vi "Asynchronous - RT Command Channels - Execute.vi"(7 "Map (RT Command Channels)":T1[](array[typedef]) {"RT Command Channel Ref" format="%.0x"}, 8 "Error (in)":errorcluster, 11 "Changes?":bool[](array[boolean])) -> (0 "Error (out)":errorcluster)   [LabVIEW 2017, in "Ballard MIL-1553 Engine.lvlib"]
uses:
  Ballard MIL-1553 Engine.lvlib
  Controls/RT Async_Map RT Command Channels.ctl
  Controls/RT Async_Map_Type.ctl
  <vilib>/NI Veristand/Custom Device API/Custom Device Item Ref.ctl
  <instrlib>/BTI1553Lib/BTI1553LV.lvlib
  <vilib>/NI VeriStand/Custom Device Tools/Custom Device Utility Library/Custom Device Utility Library.lvlib
  <vilib>/NI VeriStand/Custom Device API/Custom Device API.lvlib
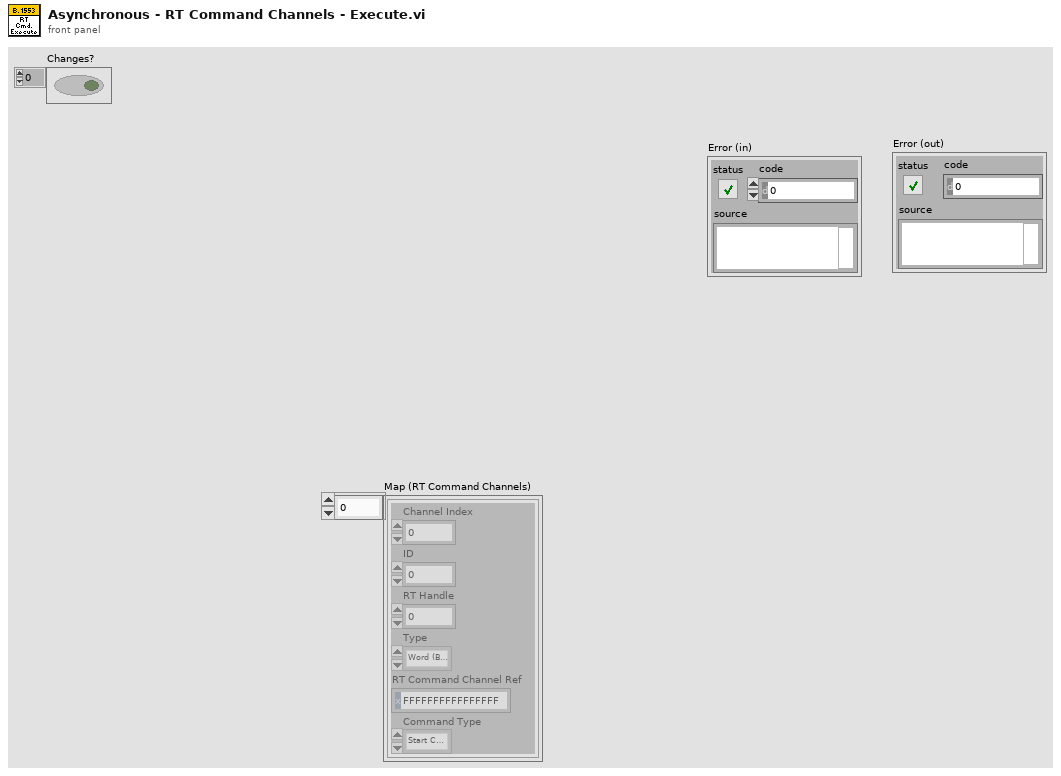
[diagram p1: front panel]
types:
  T1 = typedef "Ballard MIL-1553 Engine.lvlib/RT Async_Map RT Command Channels.ctl" = cluster{"Channel Index":i32, "ID":i32, "RT Handle":u64, "Type":T2, "RT Command Channel Ref":T3, "Command Type":enum16{"Start Command", "Stop Command"}}
  T2 = typedef "Ballard MIL-1553 Engine.lvlib/RT Async_Map_Type.ctl" = enum16{"Word (BC to RT)", "Word (MC (Rx))", "Acyclic Message Trigger", "Word (RT to ..)", "Word (RT to RT)", "Word (MC (Tx))", "RT Status", "BC Commands", "RT Commands"}
  T3 = typedef "Custom Device API.lvlib/Custom Device Item Ref.ctl" = u64
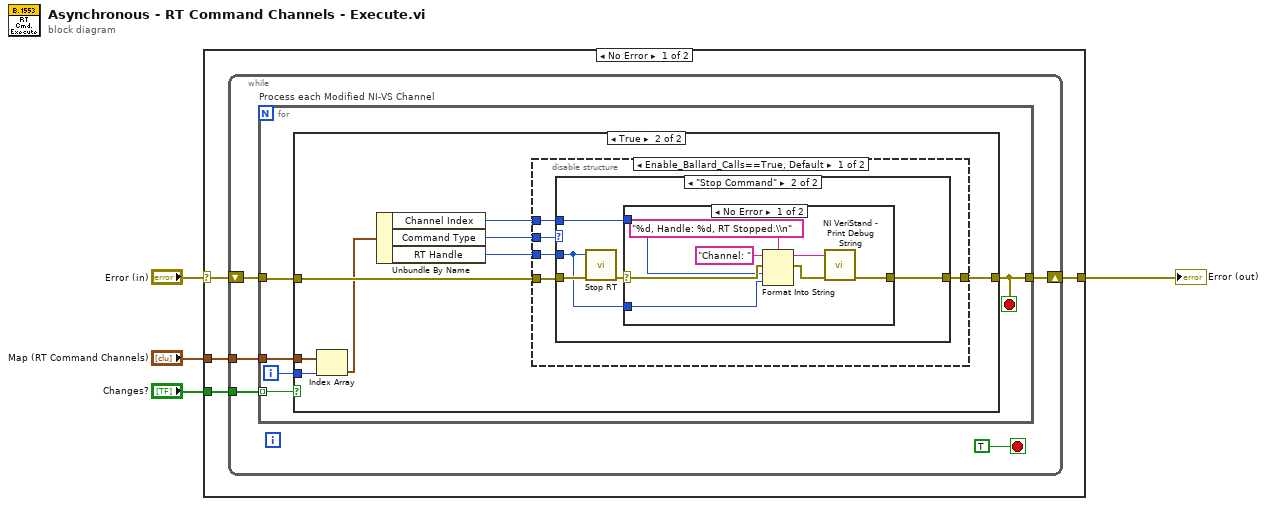
[diagram p0: block diagram]
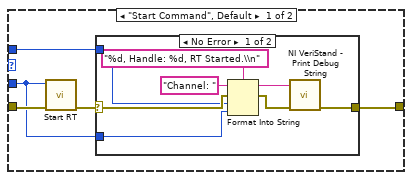
[diagram p3: hidden frame]
diagram:
  n1 = case shown="No Error" "Error (in)" {
    selector: "Error (in)" -> [w5 w62]
    tunnel: "Changes?" -> [w8 _]
    tunnel: [w7 w62] -> w3
    tunnel: "Map (RT Command Channels)" -> [w6 _]
    frame No Error {
      n2 = while {
        tunnel: w8 -> [w13]
        tunnel: w6 -> [w10]
        shift-right: [w11] -> w7
        shift-left: w5 -> [w12]
        stop <- TRUE stop-if-true
        n3 = for "Process each Modified NI-VS Channel" {
          tunnel: w13 -> [w14] mode=indexing
          tunnel: w12 -> [w18]
          tunnel: [w16] -> w11
          tunnel: w10 -> [w17]
          i -> [w15]
          stop <- w16 stop-if-true
          n4 = case shown="True" w14 {
            tunnel: w18 -> [w19 w27]
            tunnel: w17 -> [_ w26]
            tunnel: [w19 w25] -> w16
            tunnel: w15 -> [_ w24]
            frame False {
            }
            frame True {
              n5 = Index Array(array=w26, index=w24) -> (element=w23:T1)
              n6 = Unbundle By Name(w23) -> ("Channel Index"=w20:i32, "Command Type"=w22:enum16{"Start Command", "Stop Command"}, "RT Handle"=w21:u64)
              n7 = disable-structure shown="Enable_Ballard_Calls==True, Default" {
                disable-tunnel: w27 -> [w32 w61]
                disable-tunnel: [w31 w61] -> w25
                disable-tunnel: w22 -> [w30 _]
                disable-tunnel: w21 -> [w29 _]
                disable-tunnel: w20 -> [w28 _]
                frame condition #0 (active) {
                  n8 = case shown="\"Stop Command\"" w30 {
                    tunnel: w32 -> [w37 w51]
                    tunnel: [w35 w49] -> w31
                    tunnel: w29 -> [w34 w48]
                    tunnel: w28 -> [w33 w47]
                    frame "Start Command", Default {
                      n9 = call <instrlib>:"Start RT.vi"("error in (no error)"=w37, "remote terminal handle in"=w34) -> ("error out"=w36:errorcluster)  [unwired: 8 in, 1 out]
                      n10 = case shown="No Error" w36 {
                        selector: w36 -> [w40 w46]
                        tunnel: [w44 w46] -> w35
                        tunnel: w34 -> [w38 _]
                        tunnel: w33 -> [w39 _]
                        frame No Error {
                          n11 = Format Into String(format string="%d, Handle: %d, RT Started.\\n", initial string="Channel: ", error in=w40, w39, w38) -> (resulting string=w45:string, error out=w41:errorcluster)
                          n12 = call <vilib>:"NI VeriStand - Print Debug String.vi"("error in (no error)"=w41, "Message"=w45) -> ("error out"=w44:errorcluster)  [unwired: 9 in]
                        }
                        frame Error {
                        }
                      }
                    }
                    frame "Stop Command" {
                      n13 = call <instrlib>:"Stop RT.vi"("error in (no error)"=w51, "remote terminal handle in"=w48) -> ("error out"=w50:errorcluster)  [unwired: 8 in, 1 out]
                      n14 = case shown="No Error" w50 {
                        selector: w50 -> [w54 w60]
                        tunnel: [w58 w60] -> w49
                        tunnel: w48 -> [w52 _]
                        tunnel: w47 -> [w53 _]
                        frame No Error {
                          n15 = Format Into String(format string="%d, Handle: %d, RT Stopped.\\n", initial string="Channel: ", error in=w54, w53, w52) -> (resulting string=w59:string, error out=w55:errorcluster)
                          n16 = call <vilib>:"NI VeriStand - Print Debug String.vi"("error in (no error)"=w55, "Message"=w59) -> ("error out"=w58:errorcluster)  [unwired: 9 in]
                        }
                        frame Error {
                        }
                      }
                    }
                  }
                }
                frame condition #1 {
                }
              }
            }
          }
        }
      }
    }
    frame Error {
    }
  }
  "Error (out)" <- w3
